vi "open_libs.vi"(8 "error in (no error)":errorcluster, 11 "Lua in":refnum<class "Lua.lvclass">) -> (0 "error out":errorcluster, 3 "Lua out":refnum<class "Lua.lvclass">)   [LabVIEW 2020, in "Lua for LabVIEW.lvlib" / "Lua.lvclass"]
doc: "Opens all standard Lua libraries into the given state."
uses:
  Lua.lvclass
  Lua.lvclass/Lua.ctl
  lib/lua.dll/types/lua_error_code_offset.vi
  <vilib>/Utility/error.llb/Error Cluster From Error Code.vi
  lib/lua.dll/lua.dll.lvlib
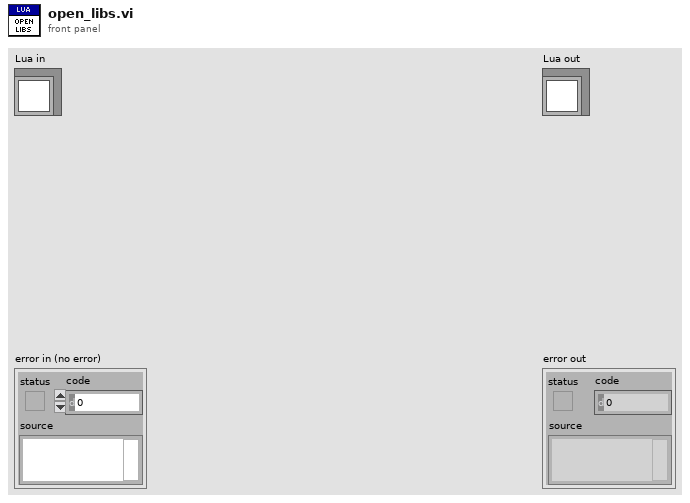
[diagram p1: front panel]
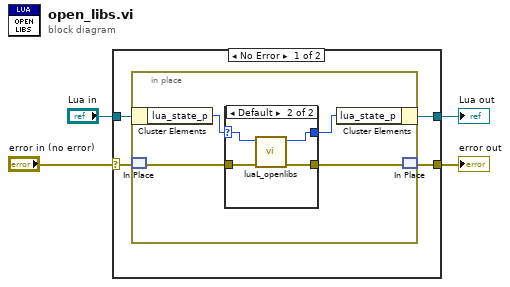
[diagram p0: block diagram]
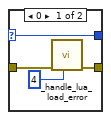
[diagram p2: hidden frame]
diagram:
  n1 = case shown="No Error" "error in (no error)" {
    selector: "error in (no error)" -> [w5 w22]
    tunnel: [w6 w22] -> w1
    tunnel: [w7 w21] -> w4
    tunnel: "Lua in" -> [w8 w21]
    frame No Error {
      n2 = in-place {
        n3 = in-place-cluster #1(w8) -> ("lua_state_p"=w11:u64)
        n4 = in-place-match #2(w5) -> (w10:errorcluster)
        n5 = case shown="Default" w11 {
          selector: w11 -> [w16 w20]
          tunnel: [w16 w19] -> w12
          tunnel: w10 -> [w13 w17]
          tunnel: [w14 w18] -> w9
          frame 0 {
            n6 = call "_handle_lua_load_error.vi"("lua_load errcode"=4, "error in (no error)"=w13) -> ("error out"=w14:errorcluster)  [unwired: 9 in]
          }
          frame Default {
            n7 = call "luaL_openlibs.vi"("error in (no error)"=w17, "lua_state_p"=w20) -> ("error out"=w18:errorcluster, "lua_state_p out"=w19:u64)  [unwired: 8 in]
          }
        }
        n8 = in-place-cluster #1("lua_state_p"=w12) -> (w7:refnum<class "Lua.lvclass">)
        n9 = in-place-match #2(w9) -> (w6:errorcluster)
      }
    }
    frame Error {
    }
  }
  "error out" <- w1
  "Lua out" <- w4
